vi "AmplitudeDetector.vi"(6 "quasi peak detector in":dbl format="%#_13g", 8 "resolution bandwidth":dbl, 9 "DetectionMode":enum16{"Peak", "Quasi Peak", "Average"}(ring), 10 "frequency":dbl, 11 "waveform":waveform(cdb)) -> (2 "valid data?":bool, 3 "Value":dbl, 4 "quasi peak detector out":dbl)   [LabVIEW 2017]
uses:
  <vilib>/Analysis/3filter.llb/Filter Passband Type.ctl
  <vilib>/Analysis/baseanly.llb/Mean (DBL).vi
  <vilib>/Analysis/5stat.llb/RMS (DBL).vi
  <vilib>/Analysis/3filter.llb/Bessel Filter (CDB).vi
  <vilib>/Analysis/NI_AALBase.lvlib
  <vilib>/Analysis/NI_AALPro.lvlib
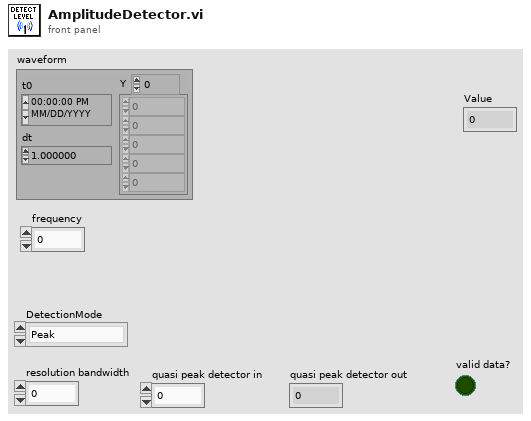
[diagram p1: front panel]
types:
  T1 = typedef "NI_AALBase.lvlib/Filter Passband Type.ctl" = enum32{"Lowpass", "Highpass", "Bandpass", "Bandstop"}
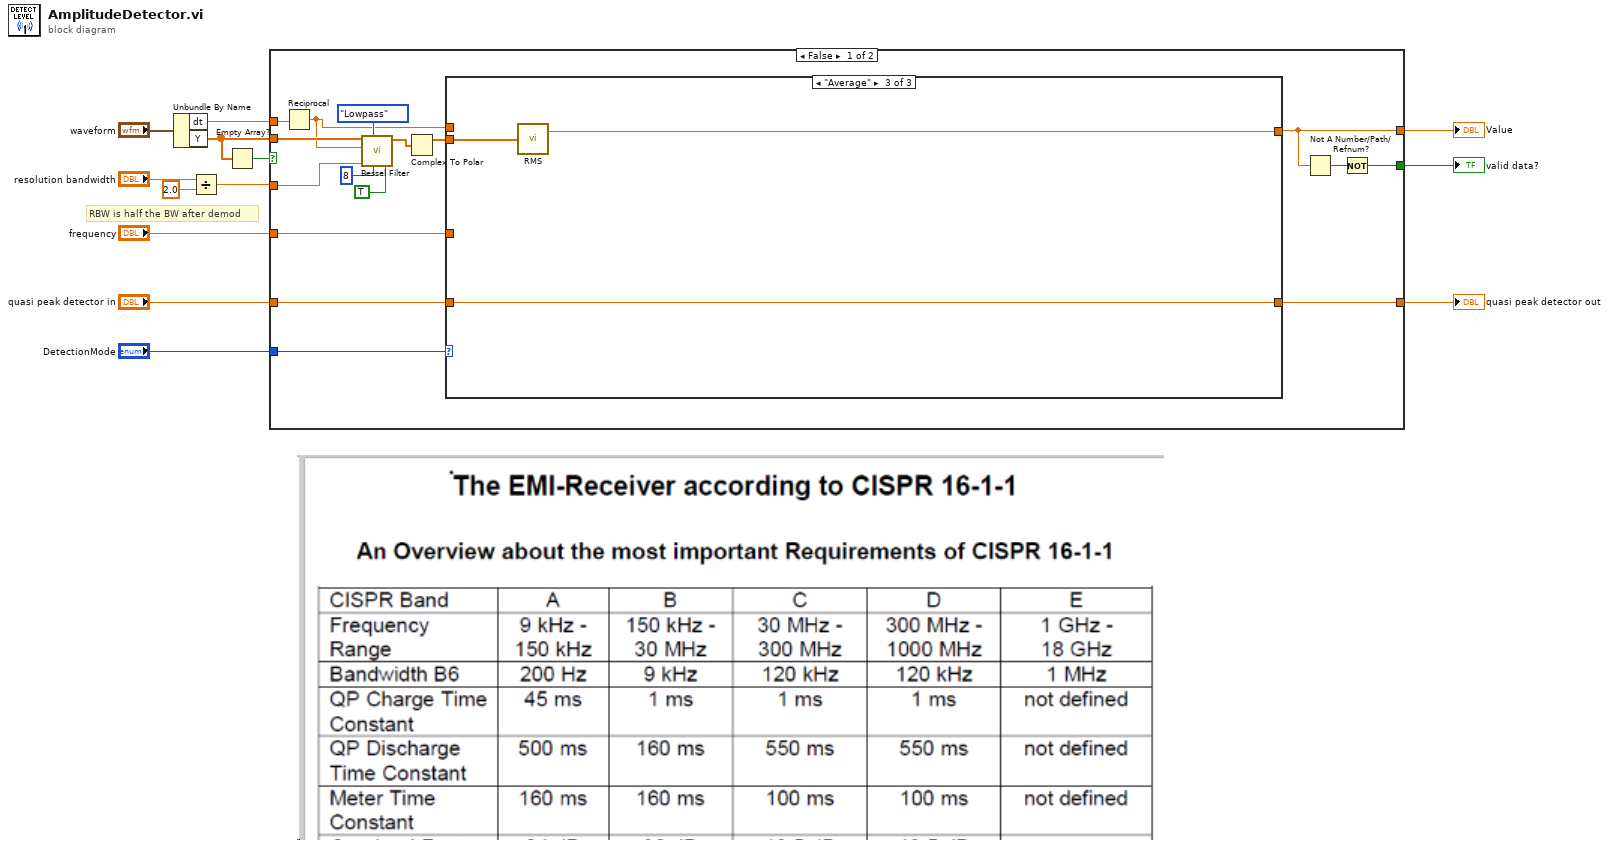
[diagram p0: block diagram]
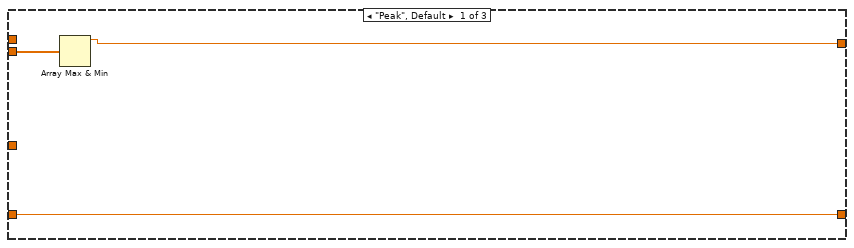
[diagram p2: hidden frame]
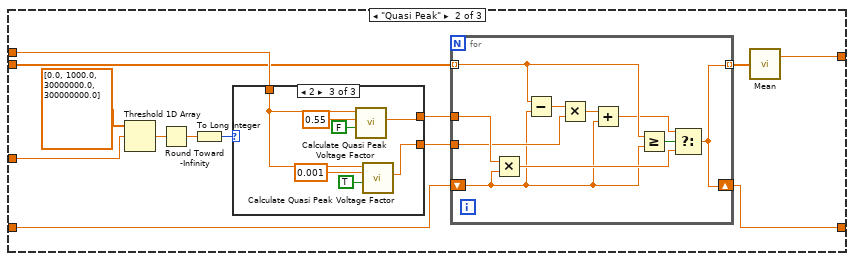
[diagram p3: hidden frame]
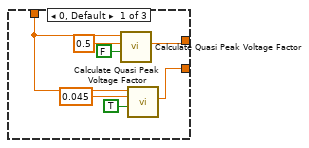
[diagram p4: hidden frame]
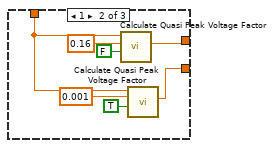
[diagram p5: hidden frame]
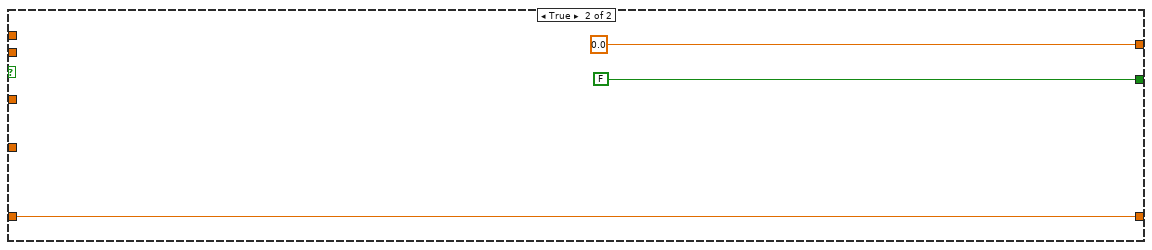
[diagram p6: hidden frame]
diagram:
  # "RBW is half the BW after demod"
  n1 = Unbundle By Name("waveform") -> ("dt"=w5:dbl, "Y"=w6:cdb[])
  n2 = Divide(x="resolution bandwidth", y=2.0) -> (x/y=w3:dbl)
  n3 = Empty Array?(array=w6) -> (empty?=w13:bool)
  n4 = case shown="False" w13 {
    tunnel: "DetectionMode" -> [w25 _]
    tunnel: [w28 sgl 0.0] -> w9
    tunnel: "frequency" -> [w29 _]
    tunnel: [w26 FALSE] -> w12
    tunnel: "quasi peak detector in" -> [w24 w80]
    tunnel: [w23 w80] -> w4
    tunnel: w6 -> [w19 _]
    tunnel: w3 -> [w18 _]
    tunnel: w5 -> [w17 _]
    frame False {
      n5 = Reciprocal(x=w17) -> (1/x=w16:dbl)
      n6 = call-poly <vilib>:"Bessel Filter.vi"("init/cont (init:F)"=TRUE, "order"=8, "filter type"=Filter_Passband_Type."Lowpass", "low cutoff freq: fl"=w18, "sampling freq: fs"=w16, "X"=w19) -> ("Filtered X"=w14:cdb[])  [unwired: 2 in, 1 out]
      n7 = Complex To Polar(r * e^(i*theta)=w14) -> (r=w15:dbl[])  [unwired: 1 out]
      n8 = case shown="\"Average\"" w25 {
        tunnel: w15 -> [w32 w34 w79]
        tunnel: [w31 w33 w77] -> w28
        tunnel: w29 -> [_ w41 _]
        tunnel: w24 -> [w30 w35 w78]
        tunnel: [w30 w37 w78] -> w23
        tunnel: w16 -> [_ w36 _]
        frame "Peak", Default {
          n9 = Array Max & Min(array=w32) -> (max value=w31:dbl)  [unwired: 3 out]
        }
        frame "Quasi Peak" {
          n10 = Threshold 1D Array(2:w41, 3:dbl[] [0.0, 1000.0, 30000000.0, 300000000.0] ("array of numbers or points")) -> (0:w44:dbl)  [unwired: 1 in]
          n11 = Round Toward -Infinity(1:w44) -> (0:w43:dbl)
          n12 = To Long Integer(number=w43) -> (32bit integer=w45:i32)
          n13 = case shown="2" w45 {
            tunnel: [w59 w66 w73] -> w40
            tunnel: [w58 w65 w72] -> w39
            tunnel: w36 -> [w62 w69 w76]
            frame 0, Default {
              n14 = call <vilib>:"Calculate Quasi Peak Voltage Factor.vi"("Charging"=FALSE, "Time Constant"=0.5, "Sample Rate"=w62) -> ("Voltage Factor"=w58:dbl)  [unwired: 8 in]
              n15 = call <vilib>:"Calculate Quasi Peak Voltage Factor.vi"("Charging"=TRUE, "Time Constant"=0.045, "Sample Rate"=w62) -> ("Voltage Factor"=w59:dbl)  [unwired: 8 in]
            }
            frame 1 {
              n16 = call <vilib>:"Calculate Quasi Peak Voltage Factor.vi"("Charging"=FALSE, "Time Constant"=0.16, "Sample Rate"=w69) -> ("Voltage Factor"=w65:dbl)  [unwired: 8 in]
              n17 = call <vilib>:"Calculate Quasi Peak Voltage Factor.vi"("Charging"=TRUE, "Time Constant"=0.001, "Sample Rate"=w69) -> ("Voltage Factor"=w66:dbl)  [unwired: 8 in]
            }
            frame 2 {
              n18 = call <vilib>:"Calculate Quasi Peak Voltage Factor.vi"("Charging"=FALSE, "Time Constant"=0.55, "Sample Rate"=w76) -> ("Voltage Factor"=w72:dbl)  [unwired: 8 in]
              n19 = call <vilib>:"Calculate Quasi Peak Voltage Factor.vi"("Charging"=TRUE, "Time Constant"=0.001, "Sample Rate"=w76) -> ("Voltage Factor"=w73:dbl)  [unwired: 8 in]
            }
          }
          n20 = for {
            tunnel: w40 -> [w49]
            tunnel: w39 -> [w55]
            tunnel: w34 -> [w51] mode=indexing
            tunnel: [w52] -> w38 mode=indexing
            shift-right: [w52] -> w37
            shift-left: w35 -> [w47]
            n21 = Multiply(x=w55, y=w47) -> (x*y=w53:dbl)
            n22 = Subtract(x=w51, y=w47) -> (x-y=w50:dbl)
            n23 = Multiply(x=w50, y=w49) -> (x*y=w48:dbl)
            n24 = Add(x=w48, y=w47) -> (x+y=w46:dbl)
            n25 = Greater Or Equal?(x=w51, y=w47) -> (x >= y?=w54:bool)
            n26 = Select(t=w46, s=w54, f=w53) -> (s? t:f=w52:dbl)
          }
          n27 = call-poly <vilib>:"Mean.vi"("X"=w38) -> ("mean"=w33:dbl)  [unwired: 1 out]
        }
        frame "Average" {
          n28 = call-poly <vilib>:"RMS.vi"("X"=w79) -> ("rms value"=w77:dbl)  [unwired: 1 out]
        }
      }
      n29 = Not A Number/Path/Refnum?(number/path/refnum=w28) -> (NaN/Path/Refnum?=w27:bool)
      n30 = Not(x=w27) -> (.not. x?=w26:bool)
    }
    frame True {
    }
  }
  "valid data?" <- w12
  "Value" <- w9
  "quasi peak detector out" <- w4
